vi "I64 to String.vi"(0 "I64":i64) -> (2 "String":string)   [LabVIEW 2011]
doc: "Convert number to string. Small VI to be block-diagram friendly.\n\nVersion 1.0 - 09/13/2013\n\nPhaeron, Inc.\nwww.phaeron.com\ninfo@phaeron.com"
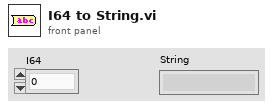
[diagram p1: front panel]
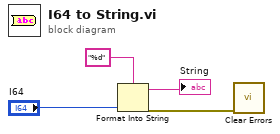
[diagram p0: block diagram]
diagram:
  n1 = Format Into String(format string="%d", "I64") -> (resulting string=→"String":string, error out=w2:errorcluster)  [unwired: 2 in]
  n2 = call <vilib>:"Clear Errors.vi"("error in (no error)"=w2) -> ()  [unwired: 6 in, 1 out]
